vi "Handle PDash UI INI Token.vi"(8 "Action":enum16{"Read", "Write", "Delete"}(ring), 11 "Use PDash UIS?":bool) -> (3 "Use PDash UIS (read)":bool)   [LabVIEW 2020, in "Panther Dashboard.lvlib"]
doc: "The intention of this VI is to\nEnable/Disable Panther Dashboard\nUIS, when Disabled, the Default\nDQMH UIs will be Used"
uses:
  Panther Dashboard.lvlib
  <resource>/dialog/lvconfig.llb/LV Config Write Boolean.vi
  <resource>/dialog/lvconfig.llb/LV Config Read Boolean.vi
panel:
  out "error out":errorcluster
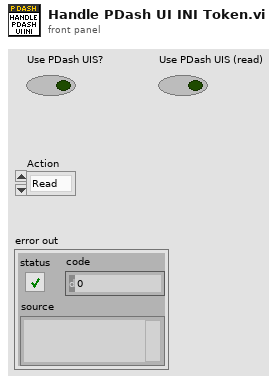
[diagram p1: front panel]
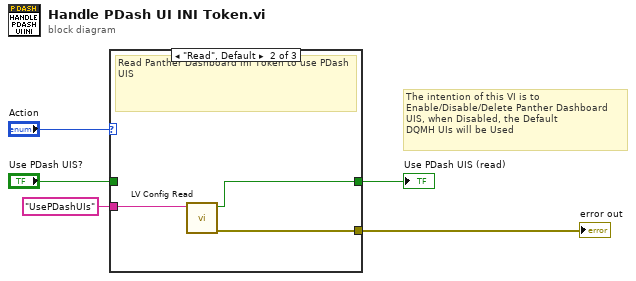
[diagram p0: block diagram]
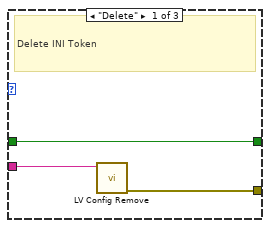
[diagram p2: hidden frame]
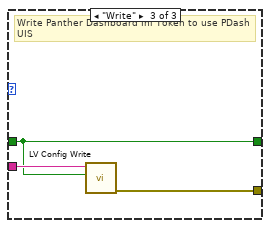
[diagram p3: hidden frame]
diagram:
  # "The intention of this VI is to\nEnable/Disable/Delete Panther Dashboard\nUIS, when Disabled, the Default\nDQMH UIs will be Used"
  n1 = case shown="\"Read\", Default" "Action" {
    tunnel: "UsePDashUIs" ("key") -> [w6 w10 w13]
    tunnel: "Use PDash UIS?" -> [w7 _ w12]
    tunnel: [w7 w9 w12] -> w2
    tunnel: [w8 w11 w14] -> w5
    frame "Delete" {
      # "Delete INI Token"
      n2 = call <resource>:"LV Config Remove.vi"("key"=w6) -> ("error out"=w8:errorcluster)  [unwired: 6 in]
    }
    frame "Read", Default {
      # "Read Panther Dashboard Ini Token to use PDash UIS"
      n3 = call-poly <resource>:"LV Config Read.vi"("key"=w10) -> ("error out"=w11:errorcluster, "value"=w9:bool)  [unwired: 4 in, 1 out]
    }
    frame "Write" {
      # "Write Panther Dashboard Ini Token to use PDash UIS"
      n4 = call-poly <resource>:"LV Config Write.vi"("value"=w12, "key"=w13) -> ("error out"=w14:errorcluster)  [unwired: 5 in]
    }
  }
  "Use PDash UIS (read)" <- w2
  "error out" <- w5
